vi "PrintMain.vi"(8 "errin":errorcluster, 11 "HTML PV path":path) -> (0 "errout":errorcluster)   [LabVIEW 2020]
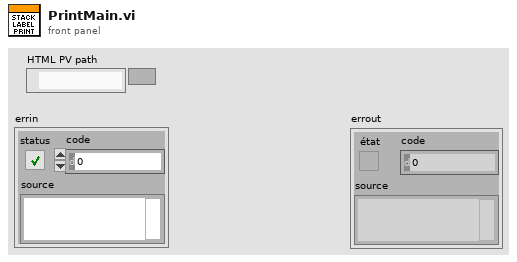
[diagram p1: front panel]
types:
  T1 = cluster{"Status":string, "SN":string, "Date test":string, "SOC":string, "Config":string}
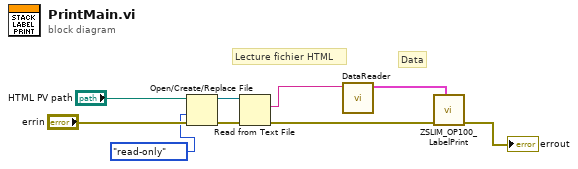
[diagram p0: block diagram]
diagram:
  # "Data"
  # "Lecture fichier HTML"
  n1 = Open/Create/Replace File(file path (use dialog)="HTML PV path", error in="errin", access (0:read/write)=enum16{"read/write", "read-only", "write-only"}."read-only") -> (refnum out=w6:refnum<file>, error out=w7:errorcluster)  [unwired: 3 in, 1 out]
  n2 = Read from Text File(file (use dialog)=w6, error in=w7) -> (text=w5:string, error out=w4:errorcluster)  [unwired: 2 in, 2 out]
  n3 = call "DataReader.vi"("PV html"=w5) -> ("Cluster"=w3:T1)  [unwired: 10 in]
  n4 = call "ZSLIM_OP100_LabelPrint.vi"("Cluster"=w3, "errin"=w4) -> ("error out"=→"errout":errorcluster)  [unwired: 9 in]
